vi "s-lab第1章 数值型数据1-7.vi"() -> ()   [LabVIEW 2013]
panel:
  out "数值 9":dbl
  out "数值 8":dbl
  out "数值 7":dbl
  in  "数值 6":dbl
  out "滑动杆 6":u8(slide) scale=0.0..10.0
  out "滑动杆 5":u8(slide) scale=0.0..10.0
  in  "滚动条 2":i32(c297)
  in  "滚动条":i32(c297)
  out "数值 f":dbl
  out "数值 c":dbl
  in  "数值 e":dbl
  in  "数值 d":dbl
  in  "数值 b":dbl
  in  "数值 a":dbl
  out "数值 5":dbl
  out "数值 4":dbl
  out "量表 2":dbl(knob) scale=0.0..10.0
  out "仪表":dbl(knob) scale=0.0..10.0
  in  "转盘":dbl(knob) scale=0.0..10.0
  in  "旋钮":dbl(knob) scale=0.0..10.0
  out "液罐":dbl(slide) scale=0.0..10.0
  out "温度计":dbl(slide) scale=0.0..100.0
  out "量表":dbl(knob) scale=0.0..10.0
  out "数值 3":dbl
  in  "滑动杆 4":dbl(slide) scale=0.0..10.0
  in  "滑动杆 3":dbl(slide) scale=0.0..100.0
  in  "滑动杆 2":dbl(slide) scale=0.0..10.0
  in  "滑动杆":dbl(slide) scale=0.0..10.0
  out "时间标识 2":timestamp
  out "数值 2":dbl
  in  "数值":dbl
  in  "时间标识":timestamp
  # "例 1"
  # "例 4"
  # "例 2"
  # "例 3"
  # "例 5"
  # "="
  # "+"
  # "*"
  # "="
  # "例 6"
  # "例 7"
  # "="
  # "-"
  # "绝对值"
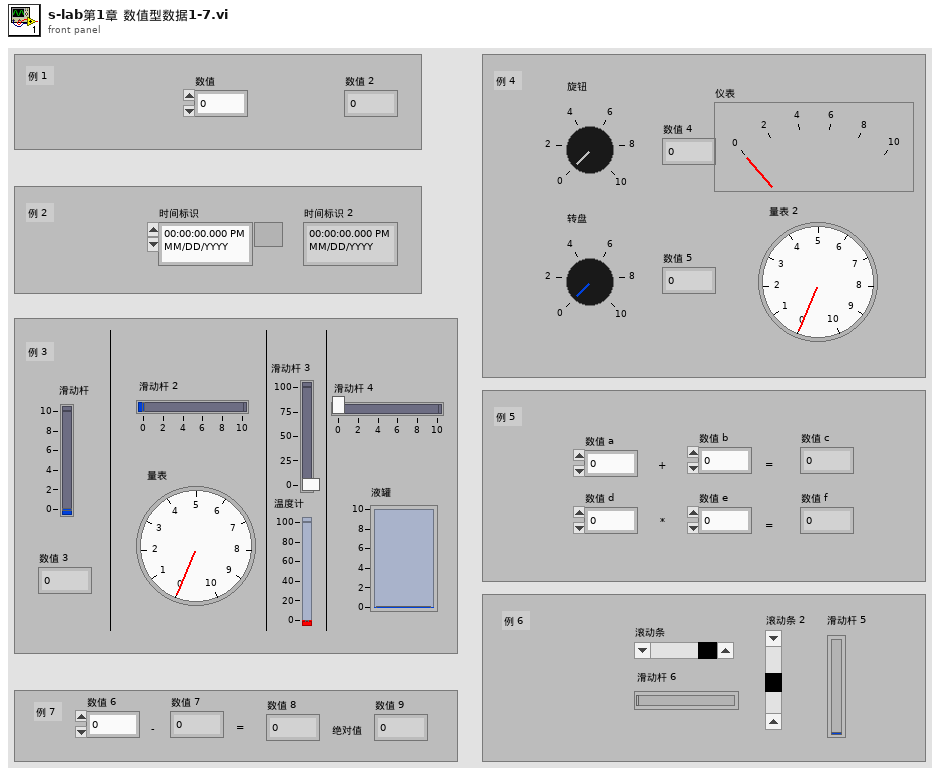
[diagram p1: front panel]
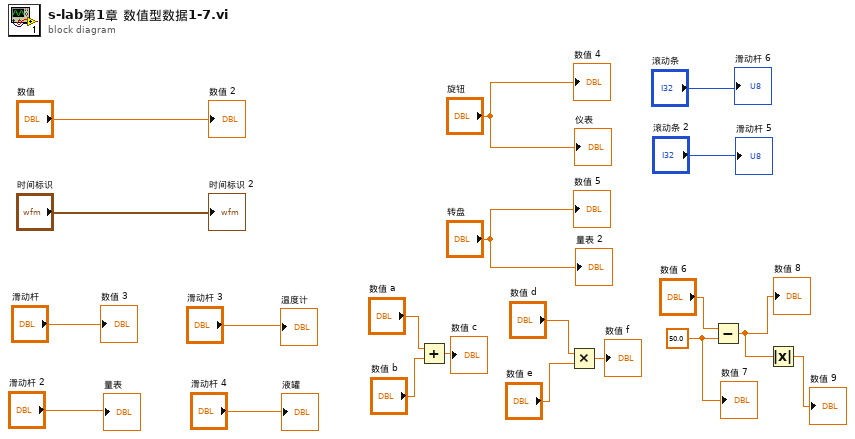
[diagram p0: block diagram]
diagram:
  w3 = 50.0 ("y")
  n1 = Add(x="数值 a", y="数值 b") -> (x+y=→"数值 c":dbl)
  n2 = Multiply(x="数值 d", y="数值 e") -> (x*y=→"数值 f":dbl)
  n3 = Subtract(x="数值 6", y=w3) -> (x-y=w1:dbl)
  "数值 8" <- w1
  n4 = Absolute Value(x=w1) -> (abs(x)=→"数值 9":dbl)
  "数值 2" <- "数值"
  "时间标识 2" <- "时间标识"
  "数值 3" <- "滑动杆"
  "量表" <- "滑动杆 2"
  "温度计" <- "滑动杆 3"
  "液罐" <- "滑动杆 4"
  "仪表" <- "旋钮"
  "量表 2" <- "转盘"
  "数值 4" <- "旋钮"
  "数值 5" <- "转盘"
  "滑动杆 5" <- "滚动条 2"
  "滑动杆 6" <- "滚动条"
  "数值 7" <- w3
